vi "Set Analog Replay Settings.vi"(8 "error in (no error)":errorcluster, 10 "Analog Replay Settings":T1 {"Voltage at max speed" min=0.0 max=10.0; "Max speed (RPM)" min=1.0; "Voltage at min speed" min=0.0 max=10.0; "Min speed (RPM)" min=0.0; "Voltage below min speed" min=0.0 max=10.0; "DAC bipolar range (V)" min=0.0001}, 11 "NodeID":u64) -> (0 "error out":errorcluster, 3 "NodeID":u64)   [LabVIEW 2015, in "Engine Simulation Toolkit Scripting API.lvlib"]
uses:
  Engine Simulation Toolkit Scripting API.lvlib
  Analog Replay Settings.ctl
  <vilib>/NI Veristand/Custom Device API/Custom Device Channel Type.ctl
  Shared/Properties.vi
  Shared/Constants and GUIDs.vi
  <vilib>/NI Veristand/Custom Device API/Set Item Property (Double).vi
  <vilib>/NI Veristand/Custom Device API/Set Item Property (Boolean).vi
  <vilib>/NI Veristand/Custom Device Tools/Custom Device Utility Library/NI VeriStand - Search for Item by Name.vi
  <vilib>/NI VeriStand/Custom Device API/Custom Device API.lvlib
  Shared/Engine Simulation Toolkit Shared.lvlib
  <vilib>/NI VeriStand/Custom Device Tools/Custom Device Utility Library/Custom Device Utility Library.lvlib
  System Explorer/Engine Simulation Toolkit System Explorer.lvlib
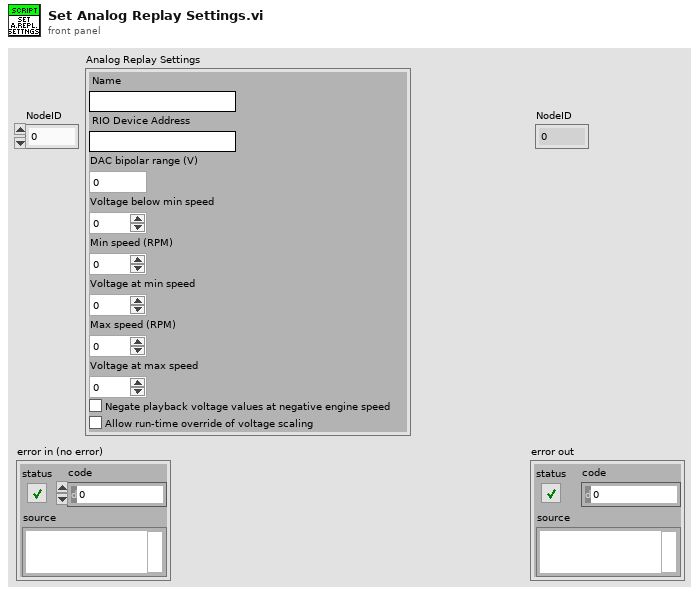
[diagram p1: front panel]
types:
  T1 = typedef "Engine Simulation Toolkit Scripting API.lvlib/Analog Replay Settings.ctl" = cluster{"Name":string, "RIO Device Address":string, "DAC bipolar range (V)":dbl, "Voltage below min speed":dbl, "Min speed (RPM)":dbl, "Voltage at min speed":dbl, "Max speed (RPM)":dbl, "Voltage at max speed":dbl, "ReverseNegate":bool, "VOverride":bool}
  T2 = typedef "Custom Device API.lvlib/Custom Device Channel Type.ctl" = enum16{"Input", "Output"}
  T3 = typedef "Custom Device API.lvlib/Custom Device Item Ref.ctl" = u64
  T4 = typedef "Engine Simulation Toolkit Shared.lvlib/Channel.ctl" = cluster{"Name":string, "Units":string, "Default":dbl, "Description":string, "Scalable":bool}
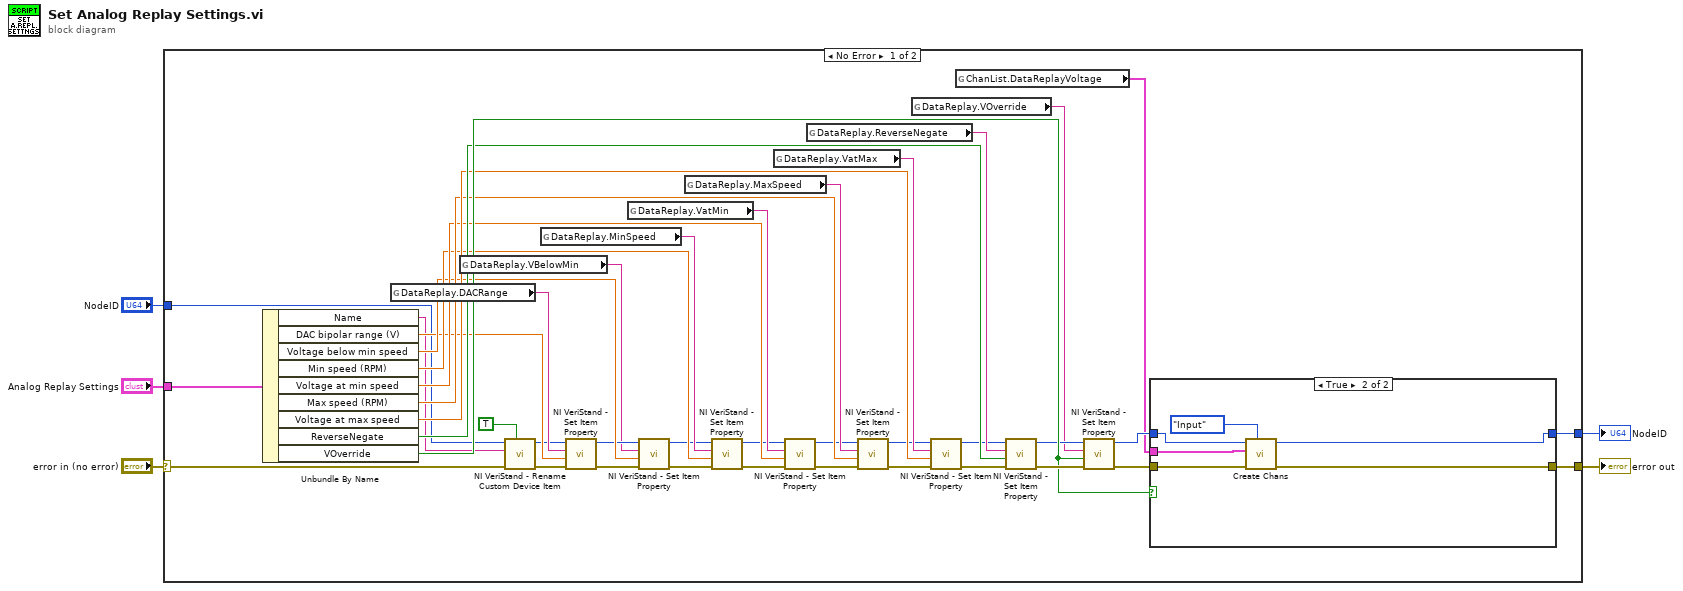
[diagram p0: block diagram]
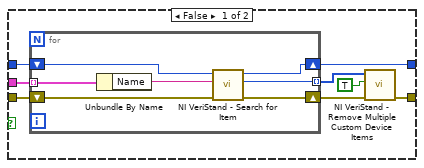
[diagram p2: hidden frame]
diagram:
  n1 = case shown="No Error" "error in (no error)" {
    selector: "error in (no error)" -> [w10 w70]
    tunnel: [w46 w70] -> w5
    tunnel: "NodeID" -> [w11 w69]
    tunnel: "Analog Replay Settings" -> [w13 _]
    tunnel: [w12 w69] -> w1
    frame No Error {
      n2 = Unbundle By Name(w13) -> ("Name"=w9:string, "DAC bipolar range (V)"=w15:dbl, "Voltage below min speed"=w19:dbl, "Min speed (RPM)"=w30:dbl, "Voltage at min speed"=w33:dbl, "Max speed (RPM)"=w35:dbl, "Voltage at max speed"=w37:dbl, "ReverseNegate"=w39:bool, "VOverride"=w43:bool)
      n3 = global read "Properties.vi" "DataReplay.DACRange"() -> (w14:string)
      n4 = global read "Properties.vi" "DataReplay.VBelowMin"() -> (w16:string)
      n5 = call <vilib>:"NI VeriStand - Rename Custom Device Item.vi"("Force Rename (F)"=TRUE, "error in (no error)"=w10, "New Name"=w9, "Item Ref in"=w11) -> ("error out"=w6:errorcluster, "Item Ref out"=w7:T3)  [unwired: 5 in, 1 out]
      n6 = global read "Properties.vi" "DataReplay.MinSpeed"() -> (w31:string)
      n7 = call-poly <vilib>:"NI VeriStand - Set Item Property.vi"("error in (no error)"=w6, "Value"=w15, "Property Name"=w14, "Item Ref in"=w7) -> ("error out"=w18:errorcluster, "Item Ref out"=w17:T3)  [unwired: 5 in, 1 out]
      n8 = global read "Properties.vi" "DataReplay.VatMin"() -> (w32:string)
      n9 = call-poly <vilib>:"NI VeriStand - Set Item Property.vi"("error in (no error)"=w18, "Value"=w19, "Property Name"=w16, "Item Ref in"=w17) -> ("error out"=w20:errorcluster, "Item Ref out"=w25:T3)  [unwired: 5 in, 1 out]
      n10 = global read "Properties.vi" "DataReplay.MaxSpeed"() -> (w34:string)
      n11 = call-poly <vilib>:"NI VeriStand - Set Item Property.vi"("error in (no error)"=w20, "Value"=w30, "Property Name"=w31, "Item Ref in"=w25) -> ("error out"=w21:errorcluster, "Item Ref out"=w26:T3)  [unwired: 5 in, 1 out]
      n12 = global read "Properties.vi" "DataReplay.VatMax"() -> (w36:string)
      n13 = call-poly <vilib>:"NI VeriStand - Set Item Property.vi"("error in (no error)"=w21, "Value"=w33, "Property Name"=w32, "Item Ref in"=w26) -> ("error out"=w22:errorcluster, "Item Ref out"=w27:T3)  [unwired: 5 in, 1 out]
      n14 = global read "Properties.vi" "DataReplay.ReverseNegate"() -> (w38:string)
      n15 = call-poly <vilib>:"NI VeriStand - Set Item Property.vi"("error in (no error)"=w22, "Value"=w35, "Property Name"=w34, "Item Ref in"=w27) -> ("error out"=w23:errorcluster, "Item Ref out"=w28:T3)  [unwired: 5 in, 1 out]
      n16 = global read "Properties.vi" "DataReplay.VOverride"() -> (w40:string)
      n17 = call-poly <vilib>:"NI VeriStand - Set Item Property.vi"("error in (no error)"=w23, "Value"=w37, "Property Name"=w36, "Item Ref in"=w28) -> ("error out"=w24:errorcluster, "Item Ref out"=w29:T3)  [unwired: 5 in, 1 out]
      n18 = global read "Constants and GUIDs.vi" "ChanList.DataReplayVoltage"() -> (w41:T4[])
      n19 = call-poly <vilib>:"NI VeriStand - Set Item Property.vi"("error in (no error)"=w24, "Value"=w39, "Property Name"=w38, "Item Ref in"=w29) -> ("error out"=w45:errorcluster, "Item Ref out"=w42:T3)  [unwired: 5 in, 1 out]
      n20 = call-poly <vilib>:"NI VeriStand - Set Item Property.vi"("error in (no error)"=w45, "Value"=w43, "Property Name"=w40, "Item Ref in"=w42) -> ("error out"=w44:errorcluster, "Item Ref out"=w47:T3)  [unwired: 5 in, 1 out]
      n21 = case shown="True" w43 {
        tunnel: w44 -> [w55 w68]
        tunnel: w47 -> [w54 w66]
        tunnel: w41 -> [w53 w65]
        tunnel: [w50 w67] -> w46
        tunnel: [w48 w63] -> w12
        frame False {
          n22 = for {
            tunnel: w53 -> [w58] mode=indexing
            shift-right: [w60] -> w52
            shift-left: w55 -> [w62]
            tunnel: [w59] -> w51 mode=indexing
            shift-right: [w56] -> w48
            shift-left: w54 -> [w61]
            n23 = Unbundle By Name(w58) -> ("Name"=w57:string)
            n24 = call-poly <vilib>:"NI VeriStand - Search for Item.vi"("error in"=w62, "Item Name"=w57, "Section Ref in"=w61) -> ("error out"=w60:errorcluster, "Item Ref"=w59:T3, "Section Ref out"=w56:T3)  [unwired: 5 in, 1 out]
          }
          n25 = call <vilib>:"NI VeriStand - Remove Multiple Custom Device Items.vi"("error in (no error)"=w52, "Force Delete (F)"=TRUE, "Item Refs in"=w51) -> ("error out"=w50:errorcluster)  [unwired: 7 in, 1 out]
        }
        frame True {
          n26 = call "Create Chans.vi"("Type"=Custom_Device_Channel_Type."Input", "error in (no error)"=w68, "Channels"=w65, "Section Ptr"=w66) -> ("error out"=w67:errorcluster, "Section Ptr dup"=w63:T3)  [unwired: 4 in, 2 out]
        }
      }
    }
    frame Error {
    }
  }
  "error out" <- w5
  "NodeID" <- w1
